vi "FTW-Test-Reflection-Datatypes.vi"() -> ()   [LabVIEW 2013]
uses:
  source/Reflection/FTW-Reflection-Types.ctl
  <vilib>/SourceControl/sccapi/SCCAPI Refnum.ctl
  <vilib>/registry/registry.llb/Registry refnum.ctl
  source/Collection/FTW-Collection-KeyValuePair.ctl
  source/actor/Message/Request/FTW-Message-IncomingRequest.lvclass
  <vilib>/FTP/ftp0.llb/FTP Session.ctl
  <vilib>/httpClient/ClientHandle.ctl
  <vilib>/SourceControl/sccapi/NI_SCC.lvlib
  <vilib>/FTP/NI_FTP.lvlib
  <vilib>/httpClient/LabVIEWHTTPClient.lvlib
panel:
  in  "DynamicData":dynamicdata(waveform)
  out "All types Passing?":bool
  out "Results Array":T2(array[cluster])
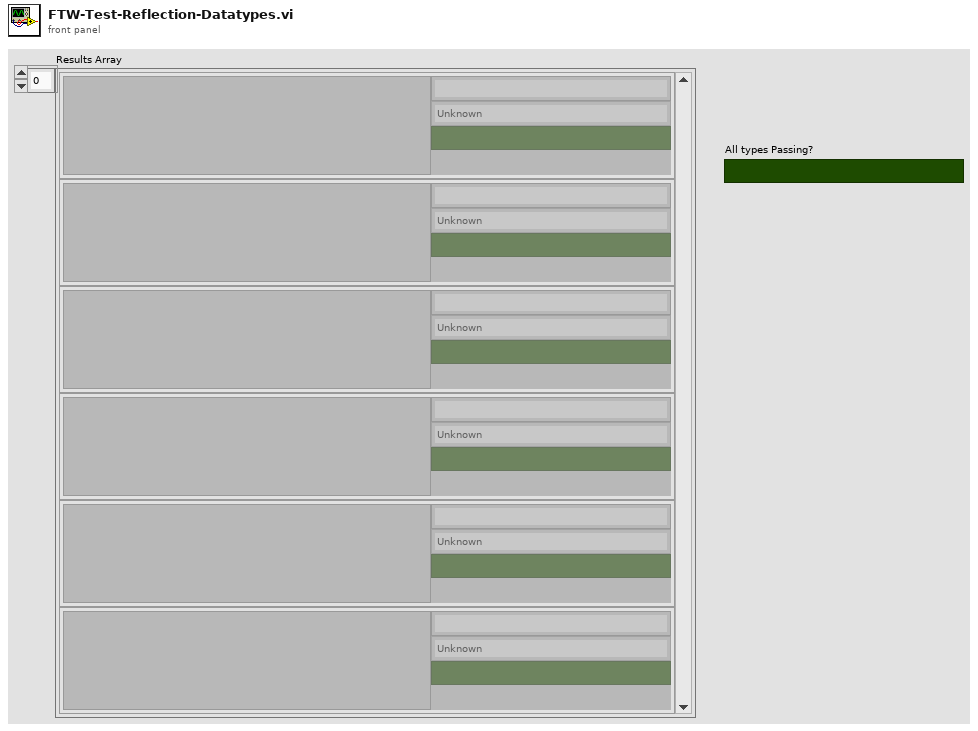
[diagram p1: front panel]
types:
  T1 = typedef "FTW-Reflection-Types.ctl" = enum16{"Unknown", "Void", "Array", "Cluster", "LVObject", "Boolean", "I8", "I16", "I32", "I64", "U8", "U16", "U32", "U64", "SGL", "DBL", "EXT", "CSG", "CDB", "CXT", "FXP", "EnumU8", "EnumU16", "EnumU32", "EnumU64", "SGLwithUnit", "DBLwithUnit", "EXTwithUnit", "CSGwithUnit", "CDBwithUnit", "CXTwithUnit", "String", "Path", "Picture", "Tag", "LVVariant", "Timestamp", "WaveformI8", "WaveformI16", "WaveformI32", "WaveformI64", "WaveformU8", "WaveformU16", "WaveformU32", "WaveformU64", "WaveformSGL", "WaveformDBL", "WaveformEXT", "WaveformCSG", "WaveformCDB", "WaveformCXT", "WaveformDigital", "WaveformUnknownType", "DigitalData", "DynamicData", "ExternalData", "FileByteStream", "TDMStream", "dotNET", "ActiveX", "VIServerReference", "VIReference", "ApplicationInstance", "Menu", "ConnectionDataSocket", "ConnectionVISA", "ConnectionBluetooth", "ConnectionIrDA", "ConnectionTCP", "ConnectionUDP", "ConnectionHTTPClient", "ConnectionFTP", "Occurrence", "Notifier", "Queue", "Rendezvous", "Semaphore", "RTFIFO", "EventPublisher", "EventRegistration", "EventCallback", "DataValueReference", "GenericClass", "GenericClassTag", "GenericClassDeepCopy", "GenericClassFlattened", "GenericClassTagFlattened", "GenericReferenceType", "WindowsRegistry", "OverloadedDatalogRef", "ReferenceUnknownType"}
  T2 = cluster{"Variant":variant, "xml string":string, "LabVIEW Type":T1, "Pass?":bool}[]
  T3 = typedef "LabVIEWHTTPClient.lvlib/ClientHandle.ctl" = refnum<k1>
  T4 = typedef "NI_FTP.lvlib/FTP Session.ctl" = refnum<k5>
  T5 = typedef "FTW-Collection-KeyValuePair.ctl" = cluster{"Key":string, "Value":string}
  T6 = typedef "Registry refnum.ctl" = refnum<k1>
  T7 = typedef "NI_SCC.lvlib/SCCAPI Refnum.ctl" = refnum<k1>
  T8 = typedef "Rendezvous RefNum" = refnum<k1>
  T9 = typedef "Semaphore RefNum" = refnum<k1>
  T10 = cluster{"Variant":variant, "Match":string, "LabVIEW Type":T1, bool}
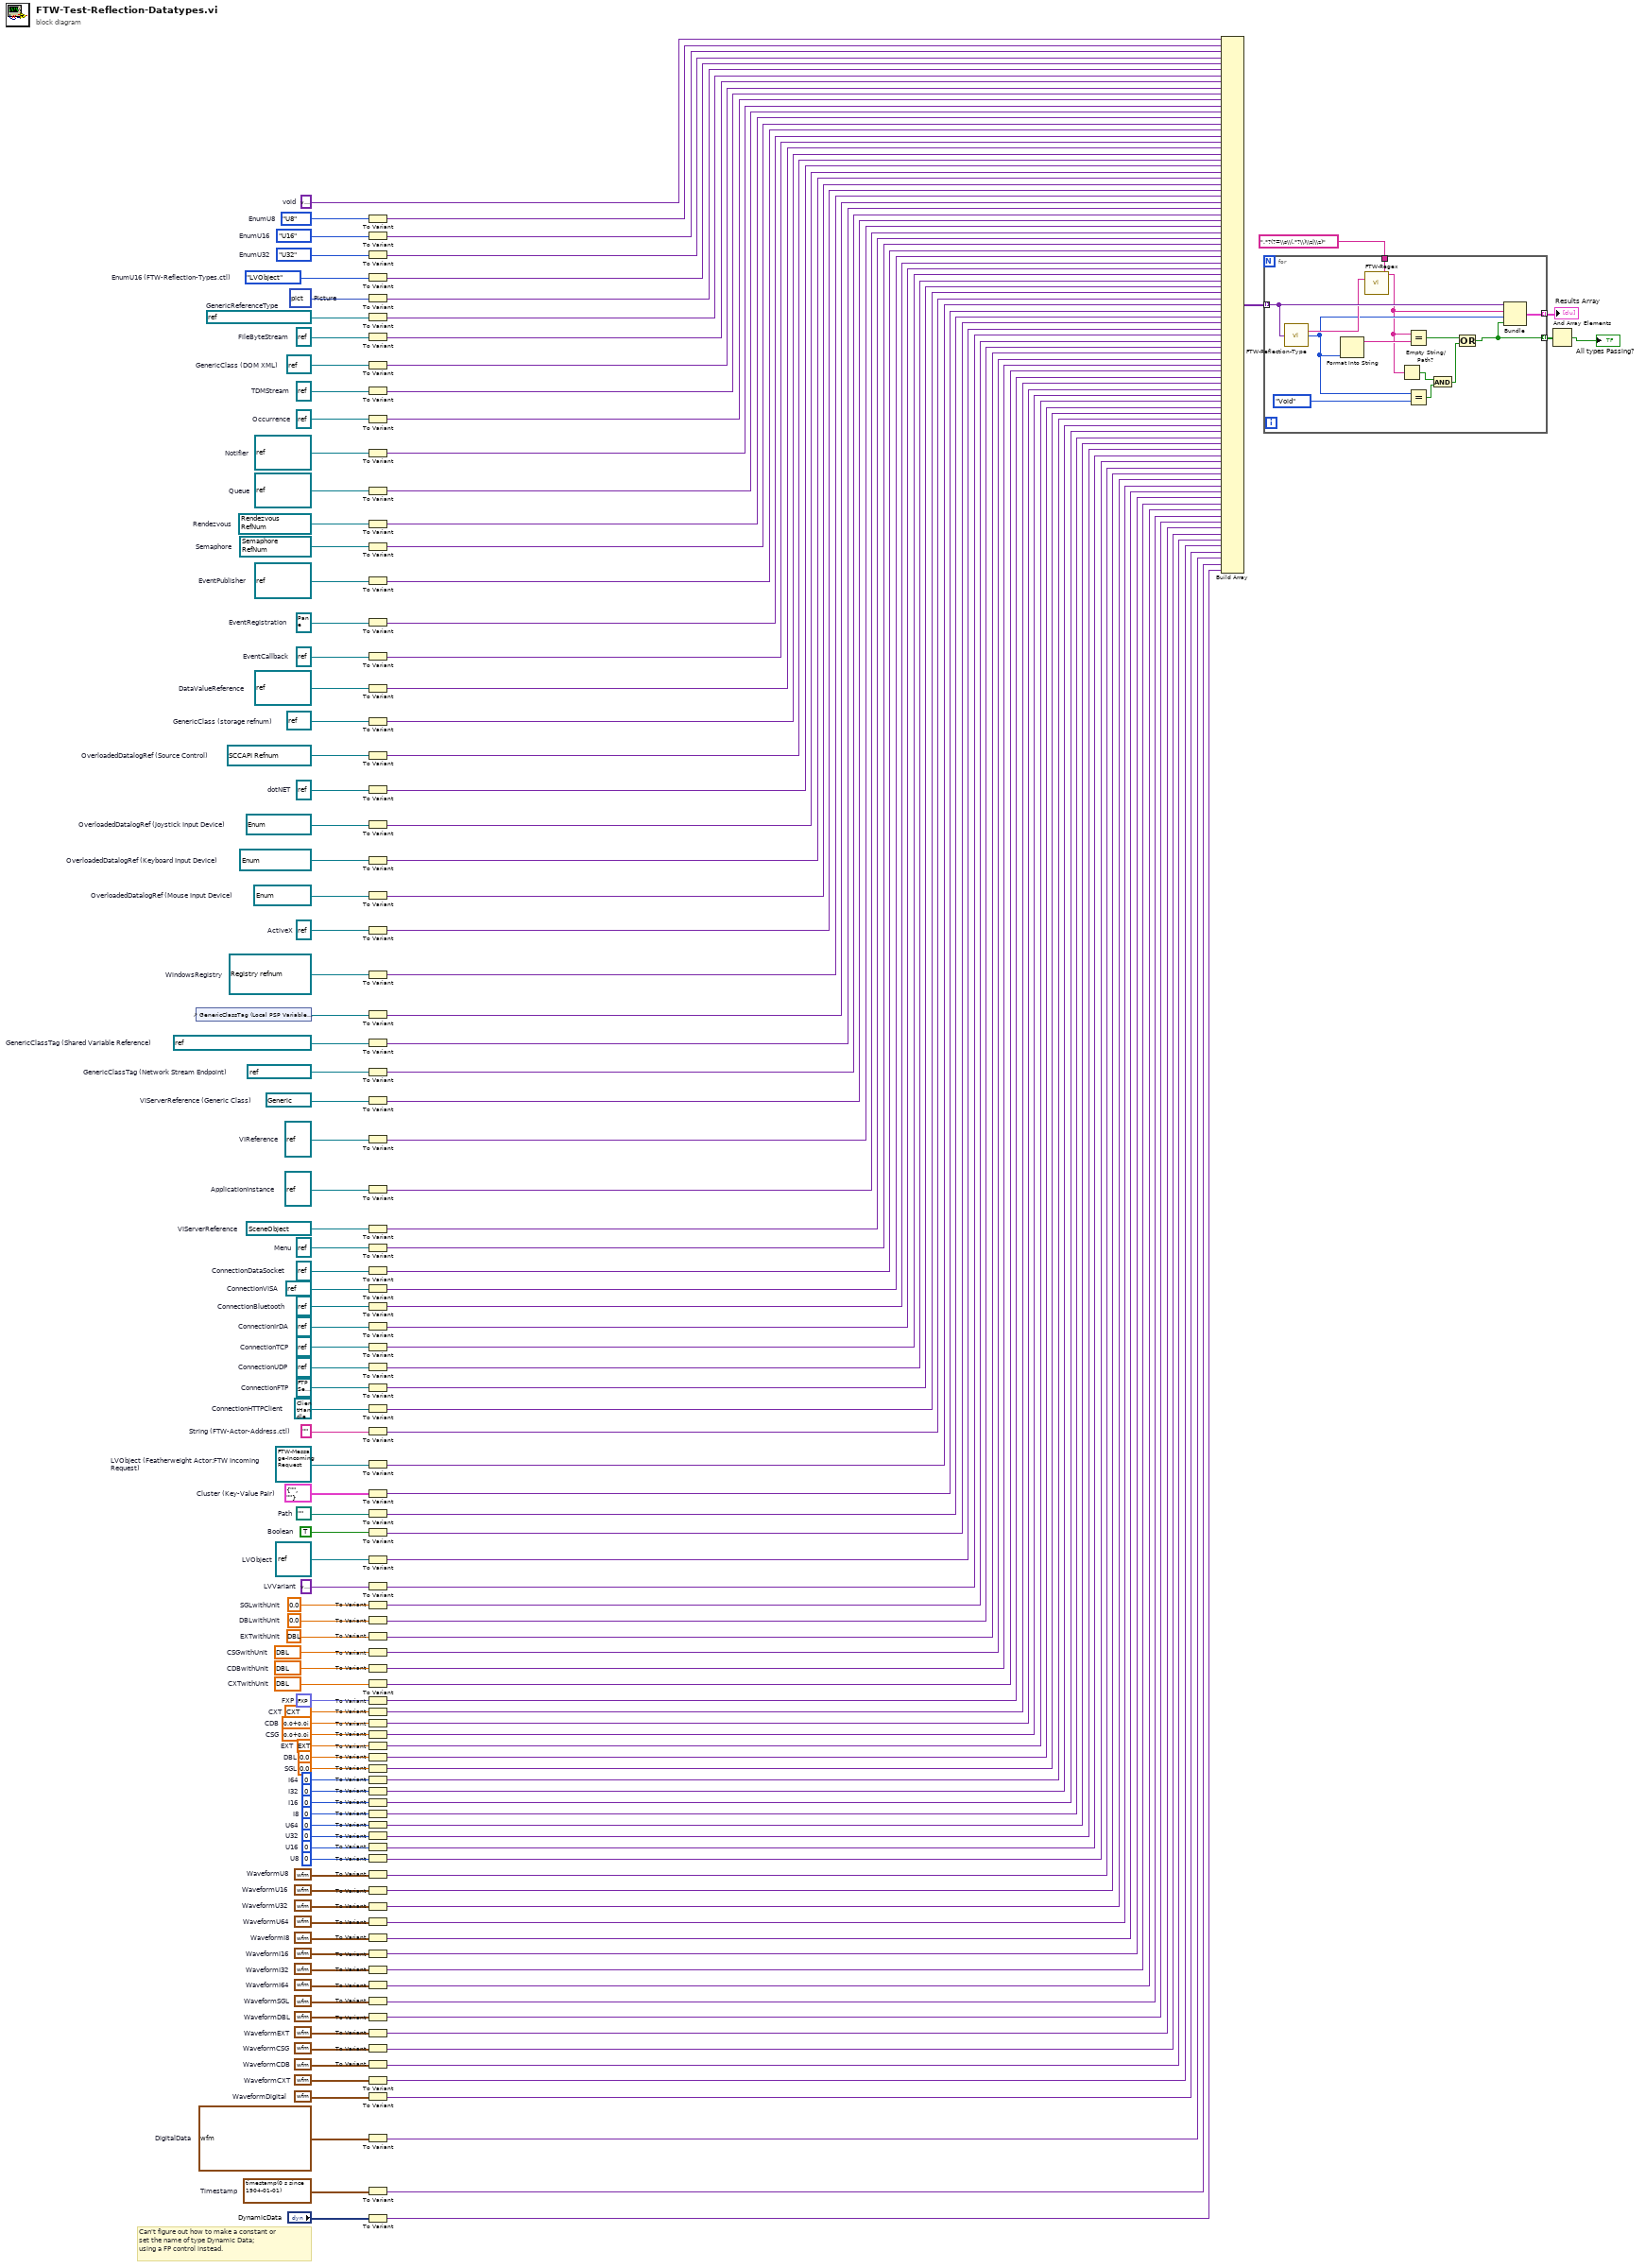
[diagram p0: block diagram]
diagram:
  w5 = digitalwaveform {"t0"=timestamp(0 s since 1904-01-01), "dt"=0.0, "Y"={"transitions"=[], "data"=[]}}  # WaveformDigital
  w6 = waveform(cxt) {"t0"=timestamp(0 s since 1904-01-01), "dt"=1.0, "Y"=[]}  # WaveformCXT
  w7 = waveform(cdb) {"t0"=timestamp(0 s since 1904-01-01), "dt"=1.0, "Y"=[]}  # WaveformCDB
  w8 = waveform(csg) {"t0"=timestamp(0 s since 1904-01-01), "dt"=1.0, "Y"=[]}  # WaveformCSG
  w9 = waveform(ext) {"t0"=timestamp(0 s since 1904-01-01), "dt"=1.0, "Y"=[]}  # WaveformEXT
  w10 = waveform(dbl) {"t0"=timestamp(0 s since 1904-01-01), "dt"=1.0, "Y"=[]}  # WaveformDBL
  w11 = waveform(sgl) {"t0"=timestamp(0 s since 1904-01-01), "dt"=1.0, "Y"=[]}  # WaveformSGL
  w12 = waveform(i64) {"t0"=timestamp(0 s since 1904-01-01), "dt"=1.0, "Y"=[]}  # WaveformI64
  w13 = waveform(i32) {"t0"=timestamp(0 s since 1904-01-01), "dt"=1.0, "Y"=[]}  # WaveformI32
  w14 = waveform(i16) {"t0"=timestamp(0 s since 1904-01-01), "dt"=1.0, "Y"=[]}  # WaveformI16
  w18 = waveform(i8) {"t0"=timestamp(0 s since 1904-01-01), "dt"=1.0, "Y"=[]}  # WaveformI8
  w19 = waveform(u64) {"t0"=timestamp(0 s since 1904-01-01), "dt"=1.0, "Y"=[]}  # WaveformU64
  w17 = waveform(u32) {"t0"=timestamp(0 s since 1904-01-01), "dt"=1.0, "Y"=[]}  # WaveformU32
  w16 = waveform(u16) {"t0"=timestamp(0 s since 1904-01-01), "dt"=1.0, "Y"=[]}  # WaveformU16
  w15 = waveform(u8) {"t0"=timestamp(0 s since 1904-01-01), "dt"=1.0, "Y"=[]}  # WaveformU8
  w21 = variant  # void
  w107 = refnum<k31> refnum  # ConnectionBluetooth
  w112 = T3 refnum  # ConnectionHTTPClient
  w64 = T4 refnum  # ConnectionFTP
  w73 = enum32{"U32"}."U32"  # EnumU32
  w72 = enum16{"U16"}."U16"  # EnumU16
  w71 = enum8{"U8"}."U8"  # EnumU8
  w111 = TRUE  # Boolean
  w116 = path ""  # Path
  w74 = FTW-Reflection-Types."LVObject"  # EnumU16 (FTW-Reflection-Types.ctl)
  w114 = refnum<class "FTW-Message-IncomingRequest.lvclass"> refnum  # LVObject (Featherweight Actor:FTW Incoming Request)
  w83 = refnum<event-registration> refnum  # EventRegistration
  w115 = T5 {"Key"="", "Value"=""}  # Cluster (Key-Value Pair)
  w113 = ""  # String (FTW-Actor-Address.ctl)
  w110 = refnum<k16> refnum  # ConnectionUDP
  w109 = refnum<k5> refnum  # ConnectionTCP
  w105 = refnum<k13> refnum  # ConnectionDataSocket
  w104 = refnum<k9> refnum  # Menu
  w87 = refnum<data-value> refnum  # DataValueReference
  w108 = refnum<k19> refnum  # ConnectionIrDA
  w75 = picture data[5B]  # Picture
  w103 = refnum<vi> refnum  # VIServerReference
  w101 = refnum<vi> refnum  # ApplicationInstance
  w102 = refnum<vi> refnum  # VIReference
  w100 = refnum<vi> refnum  # VIServerReference (Generic Class)
  w99 = refnum<k21> "localhost"  # GenericClassTag (Network Stream Endpoint)
  w88 = refnum<k27> refnum  # EventCallback
  w84 = refnum<user-event> refnum  # EventPublisher
  w80 = refnum<k4> refnum  # Occurrence
  w81 = refnum<queue> refnum  # Queue
  w82 = refnum<notifier> refnum  # Notifier
  w98 = refnum<k21> "ni.var.psp://localhost/System"  # GenericClassTag (Shared Variable Reference)
  w96 = T6 refnum  # WindowsRegistry
  w95 = refnum<k7> refnum  # ActiveX
  w94 = refnum<k1> refnum items=["MOUSE"]  # OverloadedDatalogRef (Mouse Input Device)
  w92 = refnum<k1> refnum items=["KEYBOARD"]  # OverloadedDatalogRef (Keyboard Input Device)
  w93 = refnum<k1> refnum items=["JOYSTICK"]  # OverloadedDatalogRef (Joystick Input Device)
  w89 = refnum<k24> refnum  # dotNET
  w90 = T7 refnum items=["SourceControl"]  # OverloadedDatalogRef (Source Control)
  w91 = refnum<k20> refnum  # GenericClass (storage refnum)
  w86 = T8 refnum items=["rendezvous"]  # Rendezvous
  w85 = T9 refnum items=["semaphore"]  # Semaphore
  w79 = refnum<k34> refnum  # TDMStream
  w76 = refnum<k0> refnum  # GenericReferenceType
  w106 = refnum<visa-resource-name> refnum  # ConnectionVISA
  w78 = refnum<k20> refnum  # GenericClass (DOM XML)
  w77 = refnum<file> refnum  # FileByteStream
  w118 = refnum<class> refnum  # LVObject
  w120 = variant  # LVVariant
  w132 = cxt[unit] 0.0+0.0i  # CXTwithUnit
  w131 = cdb[unit] 0.0+0.0i  # CDBwithUnit
  w130 = csg[unit] 0.0+0.0i  # CSGwithUnit
  w129 = ext[unit] 0.0  # EXTwithUnit
  w128 = dbl[unit] 0.0  # DBLwithUnit
  w127 = sgl[unit] 0.0  # SGLwithUnit
  w179 = timestamp(0 s since 1904-01-01)  # Timestamp
  w149 = cxt 0.0+0.0i  # CXT
  w150 = cdb 0.0+0.0i  # CDB
  w151 = csg 0.0+0.0i  # CSG
  w148 = fxp<+/-,64,1024> 0.0  # FXP
  w152 = ext 0.0  # EXT
  w153 = 0.0  # DBL
  w154 = sgl 0.0  # SGL
  w155 = i64 0  # I64
  w156 = 0  # I32
  w157 = i16 0  # I16
  w158 = i8 0  # I8
  w159 = u64 0  # U64
  w160 = u32 0  # U32
  w161 = u16 0  # U16
  w162 = u8 0  # U8
  w182 = digitaldata {"transitions"=[], "data"=[]}  # DigitalData
  # "Can't figure out how to make a constant or\nset the name of type Dynamic Data;\nusing a FP control instead."
  n1 = control-ref of="GenericClassTag (Local PSP Variable Engine)"() -> (w97:refnum<k21>)
  n2 = To Variant(anything=w71) -> (Variant=w23:variant)
  n3 = To Variant(anything=w72) -> (Variant=w24:variant)
  n4 = To Variant(anything=w73) -> (Variant=w25:variant)
  n5 = To Variant(anything=w74) -> (Variant=w26:variant)
  n6 = To Variant(anything=w75) -> (Variant=w27:variant)
  n7 = To Variant(anything=w76) -> (Variant=w28:variant)
  n8 = To Variant(anything=w77) -> (Variant=w29:variant)
  n9 = To Variant(anything=w78) -> (Variant=w30:variant)
  n10 = To Variant(anything=w79) -> (Variant=w31:variant)
  n11 = To Variant(anything=w80) -> (Variant=w32:variant)
  n12 = To Variant(anything=w82) -> (Variant=w33:variant)
  n13 = To Variant(anything=w81) -> (Variant=w34:variant)
  n14 = To Variant(anything=w86) -> (Variant=w35:variant)
  n15 = To Variant(anything=w85) -> (Variant=w36:variant)
  n16 = To Variant(anything=w84) -> (Variant=w37:variant)
  n17 = To Variant(anything=w83) -> (Variant=w38:variant)
  n18 = To Variant(anything=w88) -> (Variant=w39:variant)
  n19 = To Variant(anything=w87) -> (Variant=w40:variant)
  n20 = To Variant(anything=w91) -> (Variant=w41:variant)
  n21 = To Variant(anything=w90) -> (Variant=w42:variant)
  n22 = To Variant(anything=w89) -> (Variant=w43:variant)
  n23 = To Variant(anything=w93) -> (Variant=w44:variant)
  n24 = To Variant(anything=w92) -> (Variant=w45:variant)
  n25 = To Variant(anything=w94) -> (Variant=w46:variant)
  n26 = To Variant(anything=w95) -> (Variant=w47:variant)
  n27 = To Variant(anything=w96) -> (Variant=w48:variant)
  n28 = To Variant(anything=w97) -> (Variant=w49:variant)
  n29 = To Variant(anything=w98) -> (Variant=w50:variant)
  n30 = To Variant(anything=w99) -> (Variant=w51:variant)
  n31 = To Variant(anything=w100) -> (Variant=w52:variant)
  n32 = To Variant(anything=w102) -> (Variant=w53:variant)
  n33 = To Variant(anything=w101) -> (Variant=w54:variant)
  n34 = To Variant(anything=w103) -> (Variant=w55:variant)
  n35 = To Variant(anything=w104) -> (Variant=w56:variant)
  n36 = To Variant(anything=w105) -> (Variant=w57:variant)
  n37 = To Variant(anything=w106) -> (Variant=w58:variant)
  n38 = To Variant(anything=w107) -> (Variant=w59:variant)
  n39 = To Variant(anything=w108) -> (Variant=w60:variant)
  n40 = To Variant(anything=w109) -> (Variant=w61:variant)
  n41 = To Variant(anything=w110) -> (Variant=w62:variant)
  n42 = To Variant(anything=w64) -> (Variant=w63:variant)
  n43 = To Variant(anything=w112) -> (Variant=w65:variant)
  n44 = To Variant(anything=w113) -> (Variant=w66:variant)
  n45 = To Variant(anything=w114) -> (Variant=w67:variant)
  n46 = To Variant(anything=w115) -> (Variant=w68:variant)
  n47 = To Variant(anything=w116) -> (Variant=w69:variant)
  n48 = To Variant(anything=w111) -> (Variant=w70:variant)
  n49 = To Variant(anything=w118) -> (Variant=w117:variant)
  n50 = To Variant(anything=w120) -> (Variant=w119:variant)
  n51 = To Variant(anything=w127) -> (Variant=w121:variant)
  n52 = To Variant(anything=w128) -> (Variant=w122:variant)
  n53 = To Variant(anything=w129) -> (Variant=w123:variant)
  n54 = To Variant(anything=w130) -> (Variant=w124:variant)
  n55 = To Variant(anything=w131) -> (Variant=w125:variant)
  n56 = To Variant(anything=w132) -> (Variant=w126:variant)
  n57 = To Variant(anything=w148) -> (Variant=w133:variant)
  n58 = To Variant(anything=w149) -> (Variant=w134:variant)
  n59 = To Variant(anything=w150) -> (Variant=w135:variant)
  n60 = To Variant(anything=w151) -> (Variant=w136:variant)
  n61 = To Variant(anything=w152) -> (Variant=w137:variant)
  n62 = To Variant(anything=w153) -> (Variant=w138:variant)
  n63 = To Variant(anything=w154) -> (Variant=w139:variant)
  n64 = To Variant(anything=w155) -> (Variant=w140:variant)
  n65 = To Variant(anything=w156) -> (Variant=w141:variant)
  n66 = To Variant(anything=w157) -> (Variant=w142:variant)
  n67 = To Variant(anything=w158) -> (Variant=w143:variant)
  n68 = To Variant(anything=w159) -> (Variant=w144:variant)
  n69 = To Variant(anything=w160) -> (Variant=w145:variant)
  n70 = To Variant(anything=w161) -> (Variant=w146:variant)
  n71 = To Variant(anything=w162) -> (Variant=w147:variant)
  n72 = To Variant(anything=w15) -> (Variant=w178:variant)
  n73 = To Variant(anything=w16) -> (Variant=w177:variant)
  n74 = To Variant(anything=w17) -> (Variant=w176:variant)
  n75 = To Variant(anything=w19) -> (Variant=w175:variant)
  n76 = To Variant(anything=w18) -> (Variant=w174:variant)
  n77 = To Variant(anything=w14) -> (Variant=w173:variant)
  n78 = To Variant(anything=w13) -> (Variant=w172:variant)
  n79 = To Variant(anything=w12) -> (Variant=w171:variant)
  n80 = To Variant(anything=w11) -> (Variant=w170:variant)
  n81 = To Variant(anything=w10) -> (Variant=w169:variant)
  n82 = To Variant(anything=w9) -> (Variant=w168:variant)
  n83 = To Variant(anything=w8) -> (Variant=w167:variant)
  n84 = To Variant(anything=w7) -> (Variant=w166:variant)
  n85 = To Variant(anything=w6) -> (Variant=w165:variant)
  n86 = To Variant(anything=w5) -> (Variant=w164:variant)
  n87 = To Variant(anything=w182) -> (Variant=w163:variant)
  n88 = To Variant(anything=w179) -> (Variant=w22:variant)
  n89 = To Variant(anything="DynamicData") -> (Variant=w4:variant)
  n90 = Build Array(w21, w23, w24, w25, w26, w27, w28, w29, w30, w31, w32, w33, w34, w35, w36, w37, w38, w39, w40, w41, w42, w43, w44, w45, w46, w47, w48, w49, w50, w51, w52, w53, w54, w55, w56, w57, w58, w59, w60, w61, w62, w63, w65, w66, w67, w68, w69, w70, w117, w119, w121, w122, w123, w124, w125, w126, w133, w134, w135, w136, w137, w138, w139, w140, w141, w142, w143, w144, w145, w146, w147, w178, w177, w176, w175, w174, w173, w172, w171, w170, w169, w168, w167, w166, w165, w164, w163, w22, w4) -> (w180:variant[])
  n91 = for {
    tunnel: w180 -> [w194] mode=indexing
    tunnel: [w195] -> w181 mode=indexing
    tunnel: ".*?(?=\\s\\(.*?\\)\\z|\\z)" ("Regular Expression") -> [w192]
    tunnel: [w186] -> w3 mode=indexing
    n92 = call "FTW-Reflection-Type.vi"("Anything"=w194) -> ("Data Name"=w193:string, "LabVIEW Type"=w190:T1)  [unwired: 12 in, 1 out]
    n93 = Format Into String(w190) -> (resulting string=w191:string)  [unwired: 3 in, 1 out]
    n94 = call "FTW-Regex.vi"("Regular Expression"=w192, "Input String"=w193) -> ("Match"=w185:string)  [unwired: 9 in, 4 out]
    n95 = Empty String/Path?(string/path=w185) -> (empty?=w184:bool)
    n96 = Equal?(x=w185, y=w191) -> (x = y?=w187:bool)
    n97 = Equal?(x=w190, y=FTW-Reflection-Types."Void") -> (x = y?=w183:bool)
    n98 = And(x=w184, y=w183) -> (x .and. y?=w188:bool)
    n99 = Or(x=w187, y=w188) -> (x .or. y?=w186:bool)
    n100 = Bundle("Variant"=w194, "Match"=w185, "LabVIEW Type"=w190, w186) -> (w195:T10)  [unwired: 1 in]
  }
  "Results Array" <- w181
  n101 = And Array Elements(Boolean array=w3) -> (logical AND=→"All types Passing?":bool)
